vi "Read Lock-In Stream.vi"(7 "index":i32, 8 "error in":errorcluster, 10 "elements":u32=256, 11 "fpga session in":refnum<k20>) -> (0 "error out":errorcluster, 1 "read data":bool, 2 "unscaled data":i64[][](array[numeric]), 3 "fpga session out":refnum<k20>)   [LabVIEW 2017, in "Lock-In Amplifier Example Host.lvlib"]
uses:
  Lock-In Amplifier Example Host.lvlib
  fpga type.ctl
  <vilib>/Utility/error.llb/Error Cluster From Error Code.vi
  <vilib>/rvi/errors/niLvFpgaAdjustHostInterfaceError.vi
  <vilib>/rvi/interface/nirviMethod/nirviMethod.xnode
  <vilib>/FPGAPlugInAG/Dynamic/niLvFpga_ReadFifo_Dynamic.vi
  <vilib>/rvi/errors/niLvFpgaMergeErrorWithErrorCode.vi
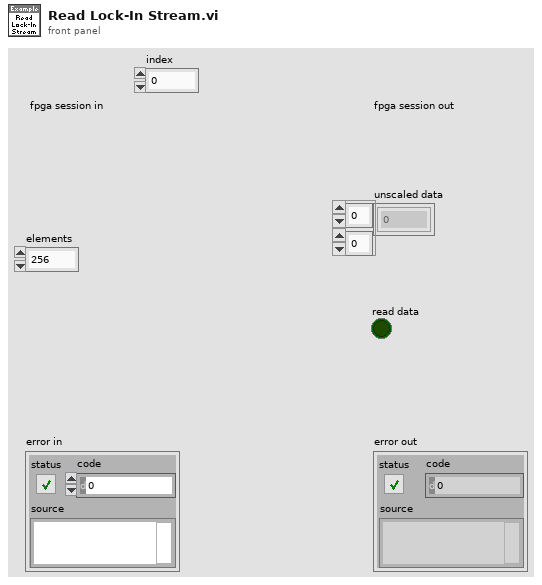
[diagram p1: front panel]
types:
  T1 = typedef "Lock-In Amplifier Example Host.lvlib/fpga type.ctl" = refnum<k20>
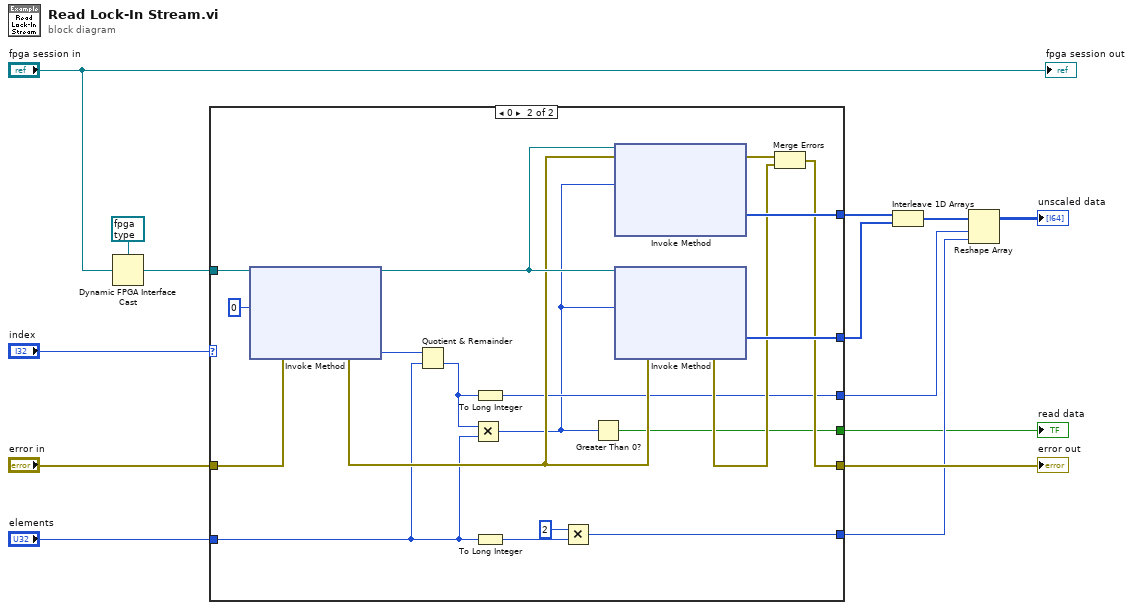
[diagram p0: block diagram]
diagram:
  n1 = Dynamic FPGA Interface Cast(Session In=T1 refnum ("fpga type"), Type="fpga session in") -> (Session Out=w12:T1)
  n2 = case shown="0" "index" {
    tunnel: w12 -> [_ w34]
    tunnel: [_ w29] -> w7
    tunnel: [_ w28] -> w6
    tunnel: "elements" -> [_ w22]
    tunnel: [_ w18] -> w3
    tunnel: "error in" -> [w15 w24]
    tunnel: [w15 w23] -> w8
    tunnel: [_ w21] -> w2
    tunnel: [_ w16] -> w1
    frame Default {
    }
    frame 0 {
      n3 = xnode "Invoke Method"("FPGA VI Reference In"=w34, "error in"=w24, "Number of Elements"=u32 0) -> ("FPGA VI Reference Out"=w31:T1, "error out"=w30:errorcluster, "Elements Remaining"=w32:u32)  [unwired: 1 in, 1 out]
      n4 = Quotient & Remainder(x=w32, y=w22) -> (floor(x/y)=w27:u32)  [unwired: 1 out]
      n5 = Multiply(x=w27, y=w22) -> (x*y=w17:u32)
      n6 = To Long Integer(number=w27) -> (32bit integer=w18:i32)
      n7 = To Long Integer(number=w22) -> (32bit integer=w19:i32)
      n8 = Multiply(x=2, y=w19) -> (x*y=w21:i32)
      n9 = Greater Than 0?(x=w17) -> (x > 0?=w16:bool)
      n10 = xnode "Invoke Method"("FPGA VI Reference In"=w31, "error in"=w30, "Number of Elements"=w17) -> ("error out"=w26:errorcluster, "Data"=w29:i64[])  [unwired: 1 in, 2 out]
      n11 = xnode "Invoke Method"("FPGA VI Reference In"=w31, "error in"=w30, "Number of Elements"=w17) -> ("error out"=w25:errorcluster, "Data"=w28:i64[])  [unwired: 1 in, 2 out]
      n12 = Merge Errors(w26, w25) -> (w23:errorcluster)
    }
  }
  "error out" <- w8
  "read data" <- w1
  n13 = Interleave 1D Arrays(w7, w6) -> (w5:i64[])
  n14 = Reshape Array(w5, w3, w2) -> (→"unscaled data":i64[][])
  "fpga session out" <- "fpga session in"
